vi "AskEventReason_UI.vi"(8 "error in (no error)":errorcluster, 10 "Event state name":string, 11 "ZenGage v3.0 UI in":refnum<class "ZenGage v3.0 UI.lvclass">) -> (0 "error out":errorcluster, 3 "ZenGage v3.0 UI out":refnum<class "ZenGage v3.0 UI.lvclass">)   [LabVIEW 2019, in "ZenGage v3.0 UI.lvclass"]
uses:
  ZenGage v3.0 UI.lvclass
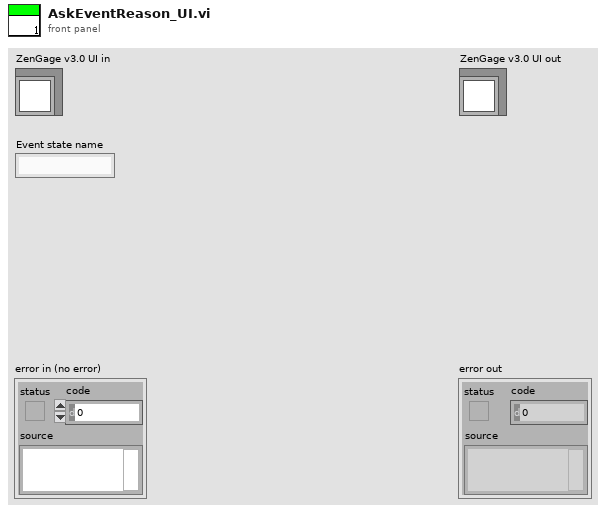
[diagram p1: front panel]
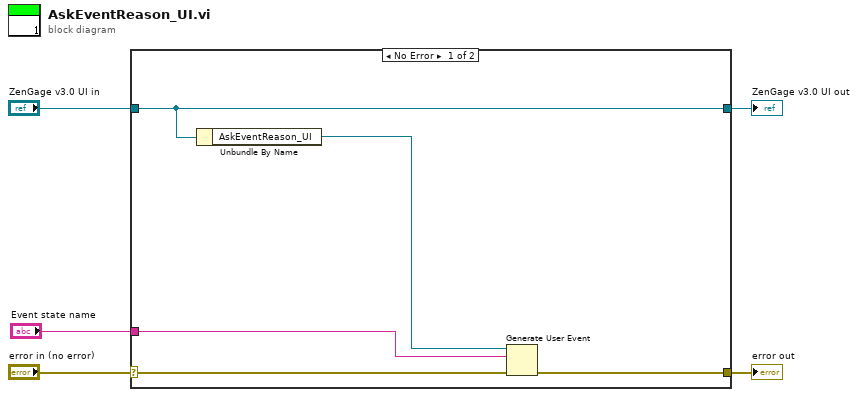
[diagram p0: block diagram]
diagram:
  n1 = case shown="No Error" "error in (no error)" {
    selector: "error in (no error)" -> [w9 w12]
    tunnel: [w8 w12] -> w4
    tunnel: [w10 w11] -> w2
    tunnel: "ZenGage v3.0 UI in" -> [w10 w11]
    tunnel: "Event state name" -> [w6 _]
    frame No Error {
      n2 = Unbundle By Name(w10) -> ("AskEventReason_UI"=w7:refnum<user-event>)
      n3 = Generate User Event(user event=w7, event data cluster=w6, error in=w9) -> (error out=w8:errorcluster)  [unwired: 1 in, 1 out]
    }
    frame Error {
    }
  }
  "error out" <- w4
  "ZenGage v3.0 UI out" <- w2
